vi "Convert Signal to Tag Bus.vi"(9 "signal mapping":T1[](array[typedef]), 10 "Signals":dbl[](array[numeric]), 11 "data table in":T3) -> (3 "data table out":T3)   [LabVIEW 2013, in "J1939.lvlib"]
uses:
  J1939.lvlib
  <vilib>/NI/Tag Bus/table/data table.ctl
  API Types/Signal Mapping.ctl
  <vilib>/NI/Tag Bus/tag/Data Type.ctl
  <vilib>/NI/Tag Bus/table/data polymorphs/write one/write Double.vi
  <vilib>/NI/Tag Bus/table/data polymorphs/write one/write Single.vi
  <vilib>/NI/Tag Bus/table/data polymorphs/write one/write I64.vi
  <vilib>/NI/Tag Bus/table/data polymorphs/write one/write I32.vi
  <vilib>/NI/Tag Bus/table/data polymorphs/write one/write I16.vi
  <vilib>/NI/Tag Bus/table/data polymorphs/write one/write I8.vi
  <vilib>/NI/Tag Bus/table/data polymorphs/write one/write U64.vi
  <vilib>/NI/Tag Bus/table/data polymorphs/write one/write U32.vi
  <vilib>/NI/Tag Bus/table/data polymorphs/write one/write U16.vi
  <vilib>/NI/Tag Bus/table/data polymorphs/write one/write U8.vi
  <vilib>/NI/Tag Bus/table/data polymorphs/write one/write Boolean.vi
  <vilib>/NI/Tag Bus/table/data table.lvlib
  <vilib>/NI/Tag Bus/tag/tag descriptor.lvclass
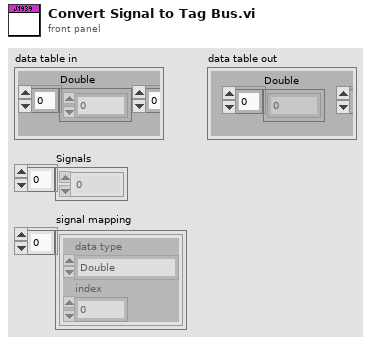
[diagram p1: front panel]
types:
  T1 = typedef "J1939.lvlib/signal mapping.ctl" = cluster{"data type":T2, "index":i32}
  T2 = typedef "tag bus.lvlib/tag descriptor.lvclass/Data Type.ctl" = enum16{"Double", "Single", "I64", "I32", "I16", "I8", "U64", "U32", "U16", "U8", "Boolean", "String", "Array of Double", "Array of Single", "Array of I64", "Array of I32", "Array of I16", "Array of I8", "Array of U64", "Array of U32", "Array of U16", "Array of U8", "Array of Boolean", "Array of String"}
  T3 = typedef "tag bus.lvlib/data table.lvlib/data table.ctl" = cluster{"Double":dbl[], "Single":sgl[], "I64":i64[], "I32":i32[], "I16":i16[], "I8":i8[], "U64":u64[], "U32":u32[], "U16":u16[], "U8":u8[], "Boolean":bool[], "String":string[], "Array of Double":cluster{"DBL Array":dbl[]}[], "Array of Single":cluster{"SGL Array":sgl[]}[], "Array of I64":cluster{"I64 Array":i64[]}[], "Array of I32":cluster{"I32 Array":i32[]}[], "Array of I16":cluster{"I16 Array":i16[]}[], "Array of I8":cluster{"I8 Array":i8[]}[], "Array of U64":cluster{"U64 Array":u64[]}[], "Array of U32":cluster{"U32 Array":u32[]}[], "Array of U16":cluster{"U16 Array":u16[]}[], "Array of U8":cluster{"U8 Array":u8[]}[], "Array of Boolean":cluster{"Boolean Array":bool[]}[], "Array of String":cluster{"String Array":string[]}[]}
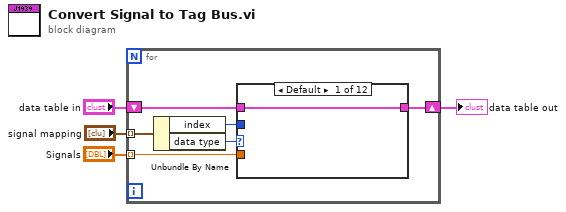
[diagram p0: block diagram]
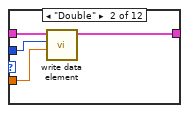
[diagram p2: hidden frame]
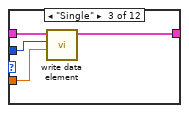
[diagram p3: hidden frame]
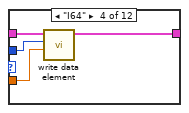
[diagram p4: hidden frame]
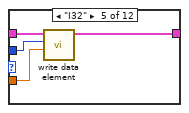
[diagram p5: hidden frame]
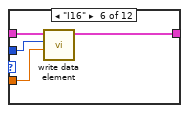
[diagram p6: hidden frame]
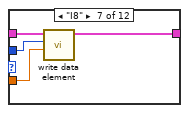
[diagram p7: hidden frame]
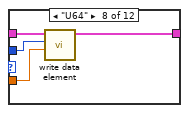
[diagram p8: hidden frame]
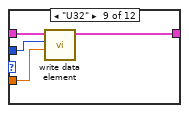
[diagram p9: hidden frame]
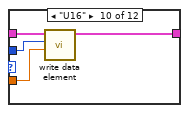
[diagram p10: hidden frame]
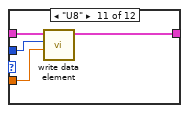
[diagram p11: hidden frame]
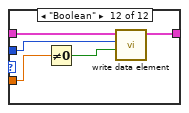
[diagram p12: hidden frame]
diagram:
  n1 = for {
    shift-right: [w8] -> w3
    shift-left: "data table in" -> [w7]
    tunnel: "signal mapping" -> [w10] mode=indexing
    tunnel: "Signals" -> [w5] mode=indexing
    n2 = Unbundle By Name(w10) -> ("index"=w6:i32, "data type"=w9:T2)
    n3 = case shown="Default" w9 {
      tunnel: [w11 w15 w19 w23 w27 w31 w35 w39 w43 w47 w51 w56] -> w8
      tunnel: w7 -> [w11 w14 w18 w22 w26 w30 w34 w38 w42 w46 w50 w55]
      tunnel: w6 -> [_ w13 w17 w21 w25 w29 w33 w37 w41 w45 w49 w54]
      tunnel: w5 -> [_ w12 w16 w20 w24 w28 w32 w36 w40 w44 w48 w53]
      frame Default {
      }
      frame "Double" {
        n4 = call-poly <vilib>:"write data element.vi"("value"=w12, "index"=w13, "data table in"=w14) -> ("data table out"=w15:T3)  [unwired: 8 in]
      }
      frame "Single" {
        n5 = call-poly <vilib>:"write data element.vi"("value"=w16, "index"=w17, "data table in"=w18) -> ("data table out"=w19:T3)  [unwired: 8 in]
      }
      frame "I64" {
        n6 = call-poly <vilib>:"write data element.vi"("value"=w20, "index"=w21, "data table in"=w22) -> ("data table out"=w23:T3)  [unwired: 8 in]
      }
      frame "I32" {
        n7 = call-poly <vilib>:"write data element.vi"("value"=w24, "index"=w25, "data table in"=w26) -> ("data table out"=w27:T3)  [unwired: 8 in]
      }
      frame "I16" {
        n8 = call-poly <vilib>:"write data element.vi"("value"=w28, "index"=w29, "data table in"=w30) -> ("data table out"=w31:T3)  [unwired: 8 in]
      }
      frame "I8" {
        n9 = call-poly <vilib>:"write data element.vi"("value"=w32, "index"=w33, "data table in"=w34) -> ("data table out"=w35:T3)  [unwired: 8 in]
      }
      frame "U64" {
        n10 = call-poly <vilib>:"write data element.vi"("value"=w36, "index"=w37, "data table in"=w38) -> ("data table out"=w39:T3)  [unwired: 8 in]
      }
      frame "U32" {
        n11 = call-poly <vilib>:"write data element.vi"("value"=w40, "index"=w41, "data table in"=w42) -> ("data table out"=w43:T3)  [unwired: 8 in]
      }
      frame "U16" {
        n12 = call-poly <vilib>:"write data element.vi"("value"=w44, "index"=w45, "data table in"=w46) -> ("data table out"=w47:T3)  [unwired: 8 in]
      }
      frame "U8" {
        n13 = call-poly <vilib>:"write data element.vi"("value"=w48, "index"=w49, "data table in"=w50) -> ("data table out"=w51:T3)  [unwired: 8 in]
      }
      frame "Boolean" {
        n14 = Not Equal To 0?(x=w53) -> (x != 0?=w52:bool)
        n15 = call-poly <vilib>:"write data element.vi"("value"=w52, "index"=w54, "data table in"=w55) -> ("data table out"=w56:T3)  [unwired: 8 in]
      }
    }
  }
  "data table out" <- w3
